vi "Buy Product.vi"(8 "error in (no error)":errorcluster, 10 "Items":string[](array[string]), 11 "Controller in":refnum<class "Controller.lvclass">) -> (0 "error out":errorcluster, 3 "Controller out":refnum<class "Controller.lvclass">)   [LabVIEW 2020, in "Controller.lvlib" / "Controller.lvclass"]
uses:
  Controller.lvclass
  Controller.lvclass/Controller.ctl
  <vilib>/ActorFramework/Message Enqueuer/Message Enqueuer.lvclass/Message Enqueuer.ctl
  Mesage Display Messages/Update Message Msg/Update Message Msg.lvclass/Update Message Msg.ctl
  <vilib>/ActorFramework/Message Enqueuer/Enqueue.vi
  Coins Messages/Reset Credit Msg/Reset Credit Msg.lvclass
  C:/Program Files (x86)/National Instruments/LabVIEW 2020/vi.lib/ActorFramework/Message/Message.lvclass
  Mesage Display Messages/Update Message Msg/Update Message Msg.lvclass
  <vilib>/ActorFramework/Message Priority Queue/Priority Enqueue.vi
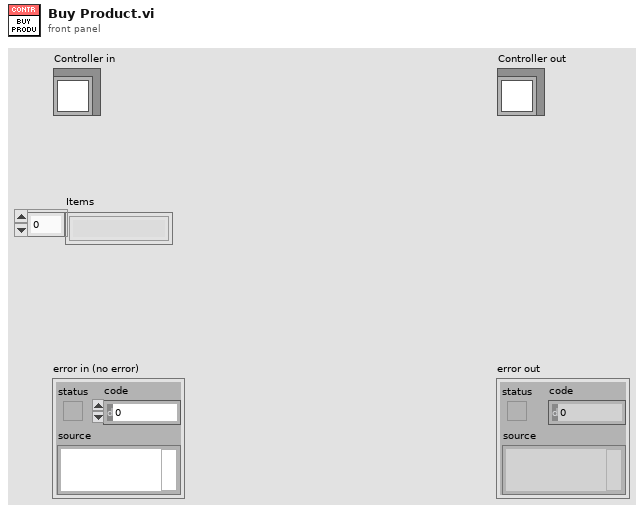
[diagram p1: front panel]
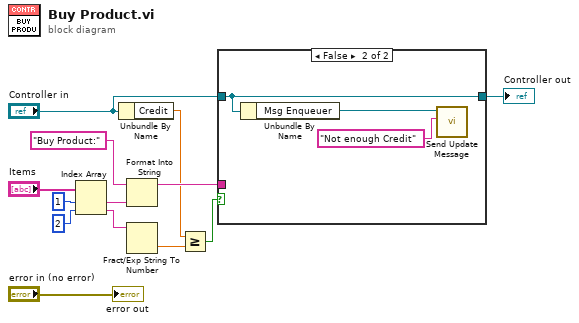
[diagram p0: block diagram]
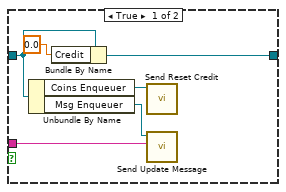
[diagram p2: hidden frame]
diagram:
  n1 = Index Array(array="Items", index #1=1 ("index"), index #2=2 ("index")) -> (element #1=w8:string, element #2=w6:string)
  n2 = Unbundle By Name("Controller in") -> ("Credit"=w5:dbl)
  n3 = Format Into String(initial string="Buy Product:" ("message"), w8) -> (resulting string=w11:string)  [unwired: 2 in, 1 out]
  n4 = Fract/Exp String To Number(string=w6) -> (number=w4:dbl)  [unwired: 3 in, 1 out]
  n5 = Greater Or Equal?(x=w5, y=w4) -> (x >= y?=w3:bool)
  n6 = case shown="False" w3 {
    tunnel: w11 -> [w16 _]
    tunnel: "Controller in" -> [w19 w22]
    tunnel: [w15 w22] -> w1
    frame True {
      n7 = Unbundle By Name(w19) -> ("Coins Enqueuer"=w18:refnum<class "Message Enqueuer.lvclass">, "Msg Enqueuer"=w17:refnum<class "Message Enqueuer.lvclass">)
      n8 = Bundle By Name(cluster=w19, "Credit"=0.0) -> (w15:refnum<class "Controller.lvclass">)
      n9 = call "Send Reset Credit.vi"("Message Enqueuer"=w18) -> ()  [unwired: 9 in, 2 out]
      n10 = call "Send Update Message.vi"("Msg"=w16, "Message Enqueuer"=w17) -> ()  [unwired: 8 in, 2 out]
    }
    frame False {
      n11 = Unbundle By Name(w22) -> ("Msg Enqueuer"=w21:refnum<class "Message Enqueuer.lvclass">)
      n12 = call "Send Update Message.vi"("Msg"="Not enough Credit", "Message Enqueuer"=w21) -> ()  [unwired: 8 in, 2 out]
    }
  }
  "Controller out" <- w1
  "error out" <- "error in (no error)"
